vi "Install Glyphs.vi"(8 "error in (no error)":errorcluster, 11 "Glyph list":T1=[{"Install"=FALSE, "Current"=bytes[272], "Icon Library"=bytes[272], "Subfolder"="", "Name"=""}]) -> (0 "error out":errorcluster)   [LabVIEW 2021]
uses:
  <resource>/plugins/NIIconEditor/Controls/IconLibraryList.ctl
  <vilib>/LabVIEW Icon API/lv_icon/Controls/Pathes.ctl
  <vilib>/LabVIEW Icon API/lv_icon/lv_icon.lvlib
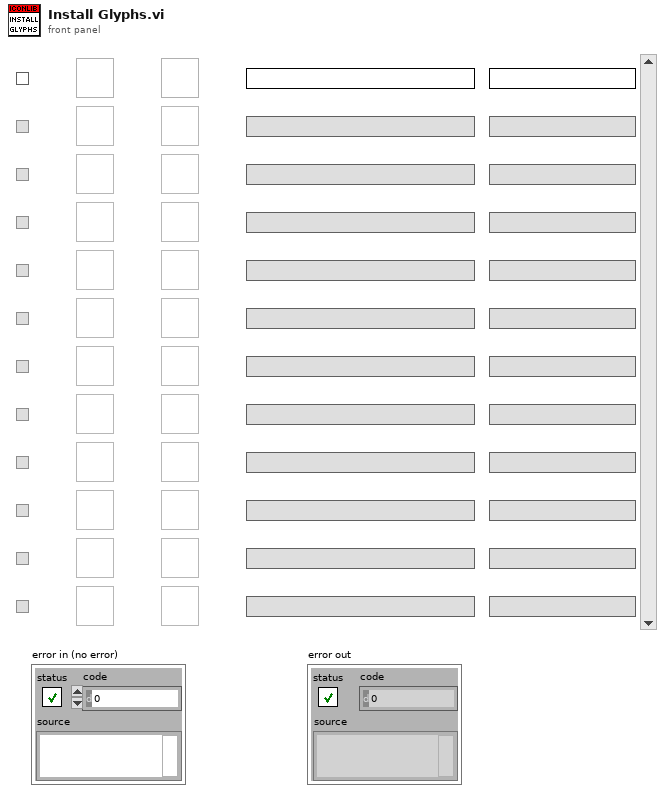
[diagram p1: front panel]
types:
  T1 = typedef "IconLibraryList.ctl" = cluster{"Install":bool, "Current":picture, "Icon Library":picture, "Subfolder":string, "Name":string}[]
  T2 = typedef "Pathes.ctl" = enum16{"Root Path", "Icon Templates", "Icon Templates VI", "Icon Templates Lib", "Glyphs"}
  T3 = typedef "imagedata.ctl" = cluster{"image type":i32, "image depth":i32, "image":u8[], "mask":u8[], "colors":u32[], "Rectangle":cluster{"left":i16, "top":i16, "right":i16, "bottom":i16}}
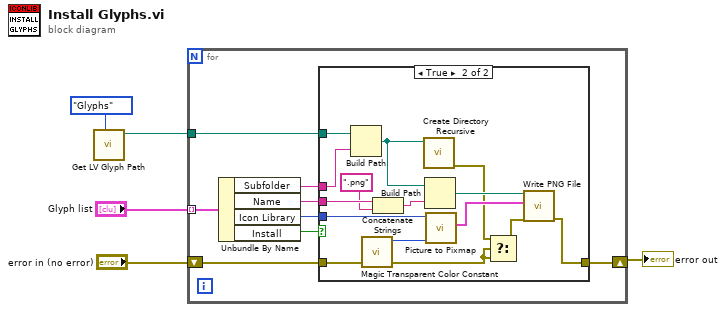
[diagram p0: block diagram]
diagram:
  n1 = call <vilib>:"Get LV Glyph Path.vi"("Path"=Pathes."Glyphs") -> ("Requested Path"=w3:path)  [unwired: 2 in, 8 out]
  n2 = for {
    tunnel: "Glyph list" -> [w13] mode=indexing
    tunnel: w3 -> [w8]
    shift-right: [w6] -> w1
    shift-left: "error in (no error)" -> [w7]
    n3 = Unbundle By Name(w13) -> ("Subfolder"=w9:string, "Name"=w10:string, "Icon Library"=w11:picture, "Install"=w12:bool)
    n4 = case shown="True" w12 {
      tunnel: w11 -> [_ w25]
      tunnel: w10 -> [_ w23]
      tunnel: w9 -> [_ w27]
      tunnel: w8 -> [_ w28]
      tunnel: w7 -> [w14 w19]
      tunnel: [w14 w20] -> w6
      frame False {
      }
      frame True {
        n5 = Build Path(base path=w28, name or relative path=w27) -> (appended path=w16:path)
        n6 = call <vilib>:"Magic Transparent Color Constant.vi"() -> ("Magic transparent color constant"=w17:u32)  [unwired: 11 out]
        n7 = Concatenate Strings(w23, ".png" ("string")) -> (w21:string)
        n8 = call <vilib>:"Create Directory Recursive.vi"("directory"=w16) -> ("error out"=w15:errorcluster)  [unwired: 2 in, 4 out]
        n9 = Build Path(base path=w16, name or relative path=w21) -> (appended path=w24:path)
        n10 = call <vilib>:"Picture to Pixmap.vi"("Background Color"=w17, "picture"=w25) -> ("image data"=w26:T3)  [unwired: 2 in, 7 out]
        n11 = Select(t=w15, s=w19, f=w19) -> (s? t:f=w18:errorcluster)
        n12 = call <vilib>:"Write PNG File.vi"("error in (no error)"=w18, "image data"=w26, "path to PNG file"=w24) -> ("error out"=w20:errorcluster)  [unwired: 8 out]
      }
    }
  }
  "error out" <- w1
